vi "KE622x -- Set Output Low Connection.vi"(0 "Resource In":refnum<visa-resource-name>, 1 "Check For SCPI Errors? (T)":bool=TRUE, 7 "Output Low Connection":T1=enum."Earth Ground", 11 "error in (no error)":errorcluster) -> (4 "Resource Out (dupl)":refnum<visa-resource-name>, 15 "error out":errorcluster)   [LabVIEW 2009, in "Keithley 622x.lvlib"]
doc: "Controls where the 'low output' of the 622x current source is connected. For the 'Earth Ground' selection, the low output is connected to the outer shield of the triax connector (note that the outer shield of the triax connector is _always_ connected to earth ground). For the 'Floating' connection, the low output is _not_ connected to the output shield (and hence not to earth ground). Instead, the low output is connected to the LO banana jack on the rear panel of the 622x. Note that via the VI named 'KE622x -- Set Triax Inner Shield Connection', it is also possible to connect the low output to the triax connector's inner shield. Note that this connection is completely independent, i.e. the low output can simulatenously connect to the triax inner shield _and_ either earth ground or the rear panel LO banana jack."
uses:
  <instrlib>/Keithley 622x LV 2009/Configure/Output/Typedefs/KE622x -- Output Low Connection.ctl
  <instrlib>/Keithley 622x LV 2009/Keithley 622x.lvlib
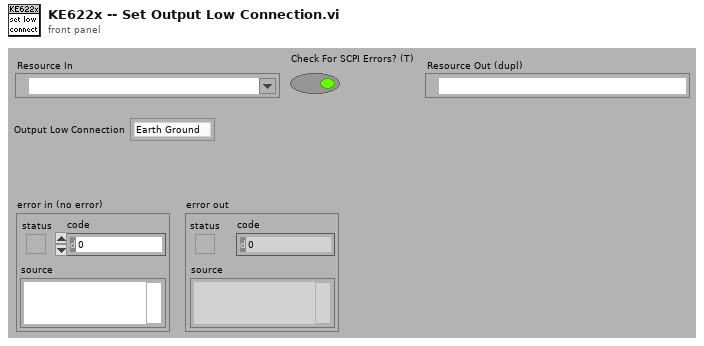
[diagram p1: front panel]
types:
  T1 = typedef "Keithley 622x.lvlib/KE622x -- Output Low Connection.ctl" = enum16{"Floating", "Earth Ground"}
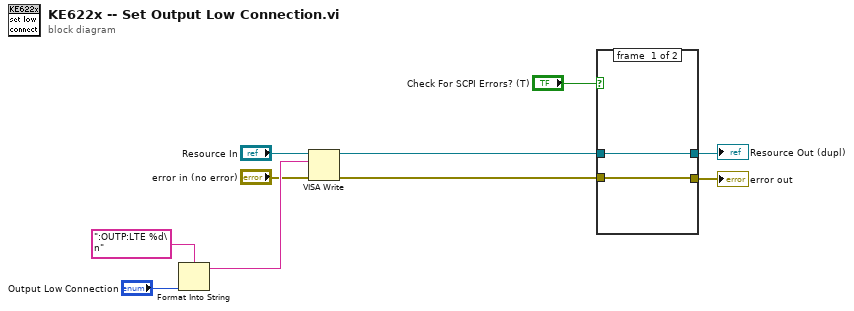
[diagram p0: block diagram]
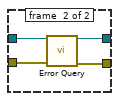
[diagram p2: hidden frame]
diagram:
  n1 = Format Into String(format string=":OUTP:LTE %d\n", "Output Low Connection") -> (resulting string=w7:string)  [unwired: 2 in, 1 out]
  n2 = VISA Write(VISA resource name="Resource In", write buffer=w7, error in (no error)="error in (no error)") -> (VISA resource name out=w4:refnum<visa-resource-name>, error out=w3:errorcluster)  [unwired: 1 out]
  n3 = case shown="False" "Check For SCPI Errors? (T)" {
    tunnel: w4 -> [w12 w16]
    tunnel: w3 -> [w11 w15]
    tunnel: [w11 w14] -> w1
    tunnel: [w12 w13] -> w2
    frame #0 {
    }
    frame #1 {
      n4 = call <instrlib>:"Error Query.vi"("VISA Resource In"=w16, "error in (no error)"=w15) -> ("VISA Resource Out (dupl)"=w13:refnum<visa-resource-name>, "error out"=w14:errorcluster)  [unwired: 10 in, 2 out]
    }
  }
  "Resource Out (dupl)" <- w2
  "error out" <- w1
